vi "Data handler-Parameter Sweep.vi"(4 "Save image":bool, 5 "Save Ref image":bool, 6 "Single Frame Data":T2, 8 "error in (no error)":errorcluster, 9 "Live graph data queue in":T1, 10 "Logging queue element in":T5={"Imaging Protocol"=enum."Live Imaging", "Number of Trials"=0, "Frame Size"=512, "# Averaged frames"=0, "Dwell time (us)"=0.0, "Index of Z-plane"=0, "Timelapse?"=FALSE, "Logging process is active"=FALSE, "Speed logging enabled"=FALSE, "tdms file ref"=refnum, "path"=path "", "Trial Number"=0, "Expected # points acquired"=FALSE, "Manually stopped"=FALSE, "Last trial"=FALSE, "Ch0 data"=[], "Ch1 data"=[], "Ref Data"=[], "Ref Frame Time"=[], "Image Time"=[], "Continuous Time"=[], "Ref X Length"=0, "Ref Y Length"=0, "# Ref Averaged frames"=0, "Ref Dwell time (us)"=0.0, "Points acquired"={"Ch0 last trial"=0, "Ch1 last trial"=0, "All trials"=0}, "HW Timings File"=refnum} {"Ref Dwell time (us)" format="%#.6g"; "Frame Size" items=["100X100"=100, "128X128"=128, "200X200"=200, "256X256"=256, "512X512"=512, "1024x1024"=1024, "2048x2048"=2048]; "Dwell time (us)" format="%#.6g"}, 11 "Image array":T3) -> (0 "error out":errorcluster)   [LabVIEW 2017]
uses:
  Typedefs/Logging queue element.ctl
  Typedefs/Imaging Protocols enum.ctl
  Typedefs/Frame Size.ctl
  Typedefs/Acquired points count.ctl
  User Interface/Queue/Live graphs queue/Typedefs/Live imaging queue element.ctl
  <vilib>/vision/Image Controls.llb/IMAQ Image.ctl
  Typedefs/Frame data dual cluster.ctl
  User Interface/Typedefs/Live graph data queue ref.ctl
  Typedefs/fgv_actions.ctl
  Typedefs/Subpanel close request.ctl
  Typedefs/Top level VI states.ctl
  Typedefs/Channel Selector.ctl
  Global Variables/General Globals.vi
panel:
  out "Subpanel is closed / Proceed":bool
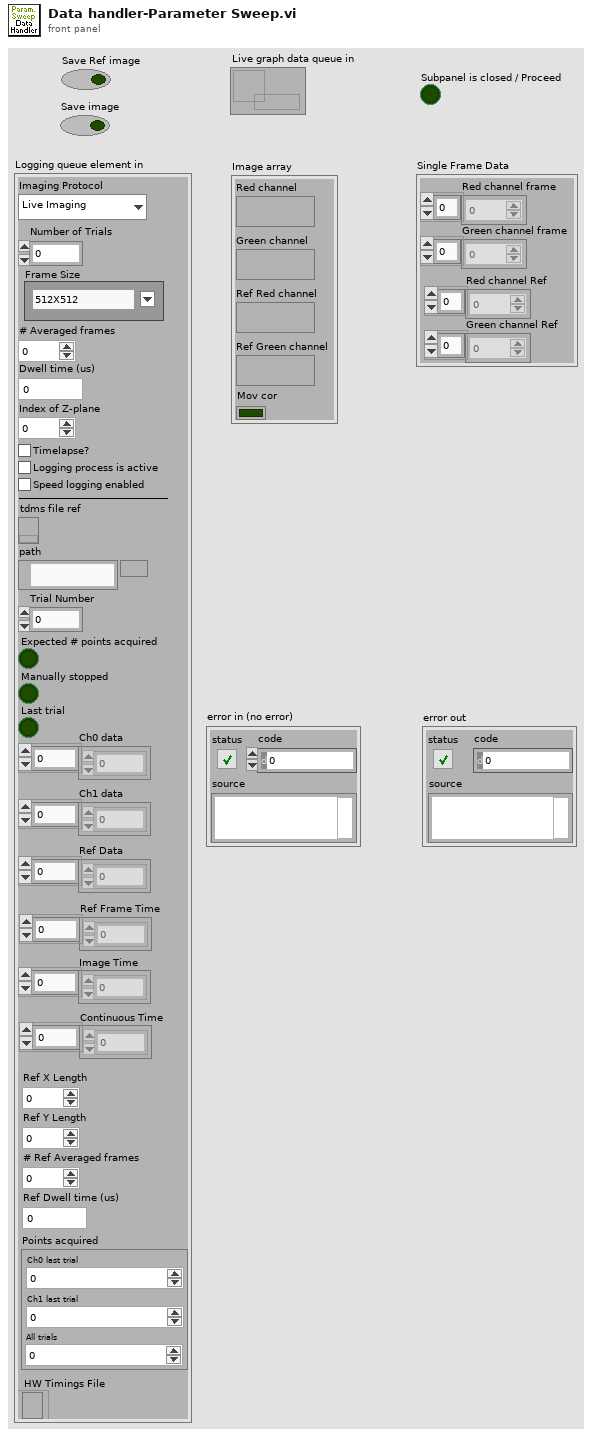
[diagram p1: front panel]
types:
  T1 = typedef "Live graph data queue ref.ctl" = refnum<queue>
  T2 = typedef "Frame data dual cluster.ctl" = cluster{"Red channel frame":dbl[], "Green channel frame":dbl[], "Red channel Ref":dbl[], "Green channel Ref":dbl[]}
  T3 = typedef "Live imaging queue element.ctl" = cluster{"Red channel":T4, "Green channel":T4, "Ref Red channel":T4, "Ref Green channel":T4, "Mov cor":bool}
  T4 = typedef "IMAQ Image.ctl" = refnum<image>
  T5 = typedef "Logging queue element.ctl" = cluster{"Imaging Protocol":T6, "Number of Trials":u16, "Frame Size":T7, "# Averaged frames":u16, "Dwell time (us)":dbl, "Index of Z-plane":i32, "Timelapse?":bool, "Logging process is active":bool, "Speed logging enabled":bool, "tdms file ref":refnum<k34>, "path":path, "Trial Number":i32, "Expected # points acquired":bool, "Manually stopped":bool, "Last trial":bool, "Ch0 data":u32[], "Ch1 data":u32[], "Ref Data":u32[], "Ref Frame Time":u64[], "Image Time":u64[], "Continuous Time":u64[], "Ref X Length":u16, "Ref Y Length":u16, "# Ref Averaged frames":u16, "Ref Dwell time (us)":dbl, "Points acquired":T8, "HW Timings File":refnum<file>}
  T6 = typedef "Imaging Protocols enum.ctl" = enum16{"AOL Z-Stack", "Motor Z Stack", "Parameter Sweep", "Functional Acquisition", "Single Plane Acquisition", "Volume Acquisition", "Live Imaging", "Live Plane Imaging", "Live Volume Imaging"}
  T7 = typedef "Frame Size.ctl" = u16
  T8 = typedef "Acquired points count.ctl" = cluster{"Ch0 last trial":u64, "Ch1 last trial":u64, "All trials":u64}
  T9 = typedef "fgv_actions.ctl" = enum16{"Get", "Set"}
  T10 = typedef "Subpanel close request.ctl" = enum16{"Request subpanel close", "Just check subpanel is closed"}
  T11 = typedef "Top level VI states.ctl" = enum16{"None", "Initialise UI", "<STACK PROTOCOL STATES>", "AOL Zstack-START", "AOL Zstack-STOP", "Motor Zstack-START", "Motor Zstack-STOP", "Parameter Sweep-START", "Parameter Sweep-STOP", "<ACQUISITION PROTOCOL STATES> ", "Functional Acquisition-START", "Functional Acquisition-STOP", "Single Plane Acquisition-START", "Single Plane Acquisition-STOP", "Volume Acquisition-START", "Volume Acquisition-STOP", "<LIVE IMAGING PROTOCOL STATES>", "Live Imaging-START", "Live Imaging-STOP", "Live Plane Imaging-START", "Live Plane Imaging-STOP", "Live Volume Imaging-START", "Live Volume Imaging-STOP", "<MOVEMENT CORRECTION PROTOCOL STATES>", "EXIT"}
  T12 = enum16{"open", "replace", "create", "open or create", "replace or create", "replace or create with confirmation"}
  T13 = typedef "Channel Selector.ctl" = enum16{"Red Channel", "Green Channel", "Blended"}
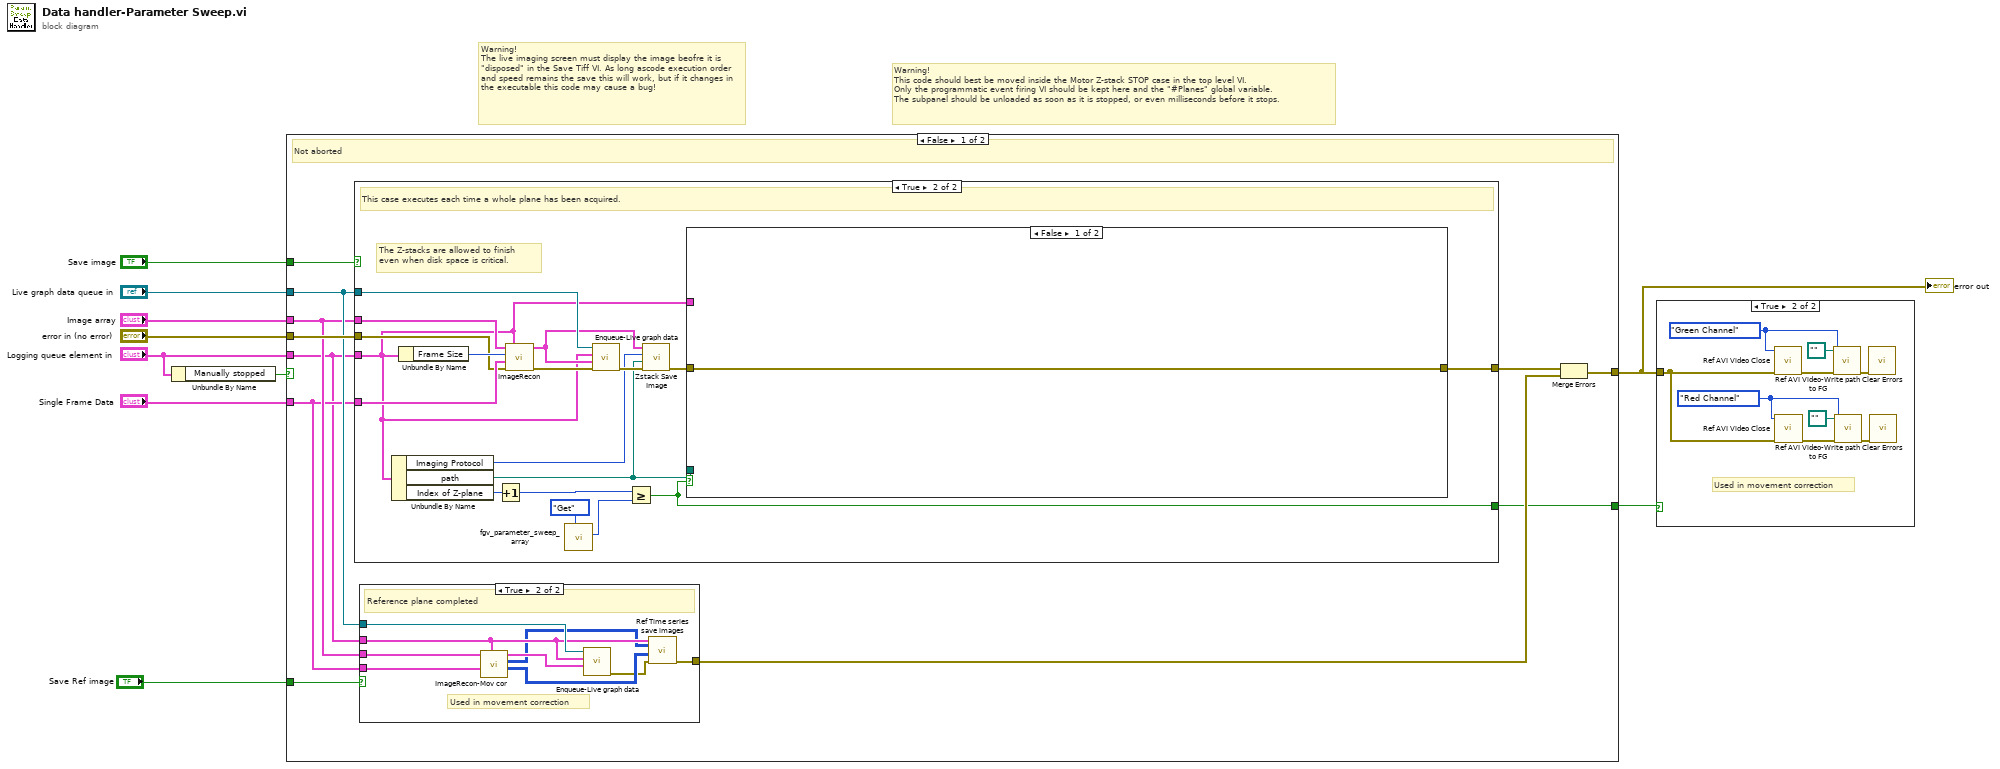
[diagram p0: block diagram]
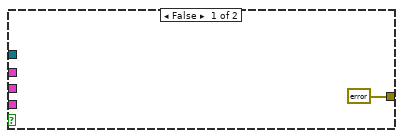
[diagram p2: hidden frame]
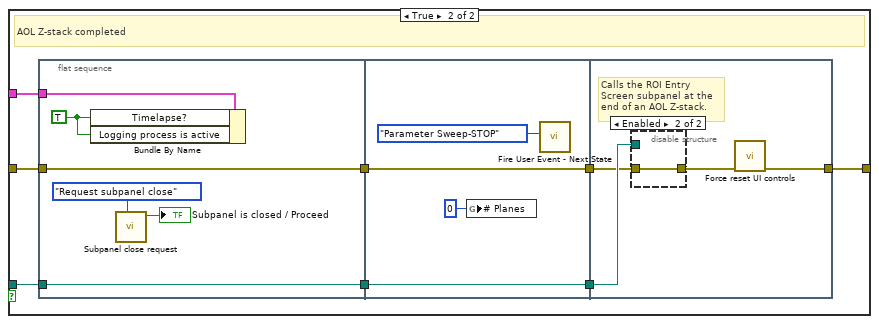
[diagram p4: hidden frame]
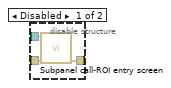
[diagram p5: hidden frame]
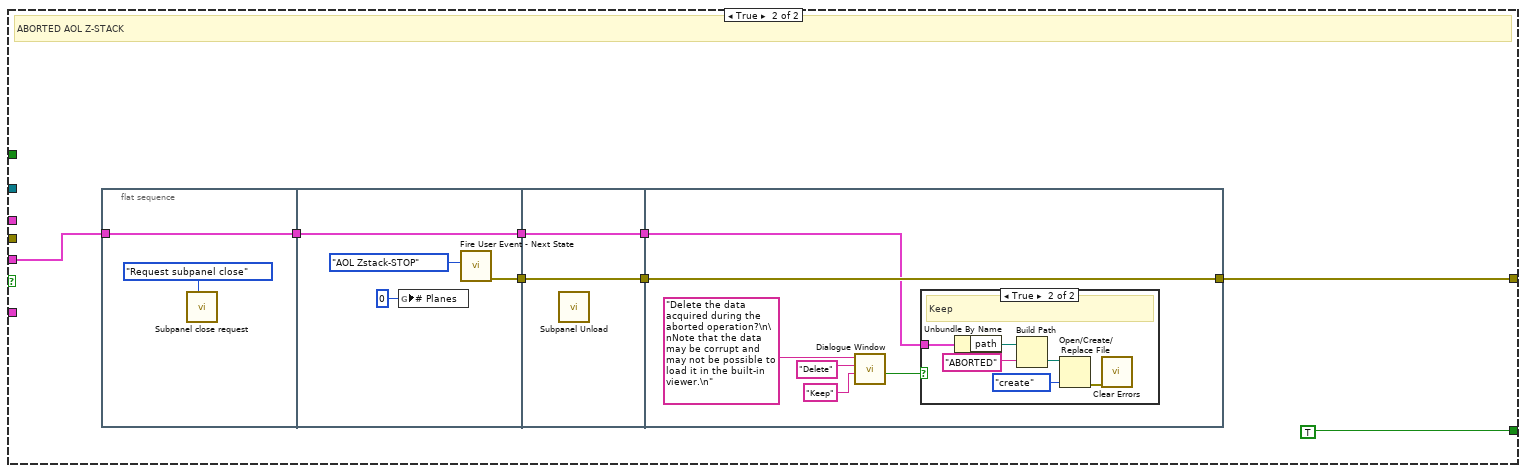
[diagram p6: hidden frame]
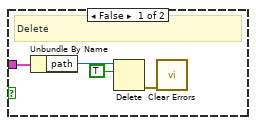
[diagram p7: hidden frame]
diagram:
  # "Warning!\nThe live imaging screen must display the image beofre it is \"disposed\" in the Save Tiff VI. As long ascode execution order and speed remains the save this will work, but if it changes in the executable this code may cause a bug!"
  # "Warning!\nThis code should best be moved inside the Motor Z-stack STOP case in the top level VI.\nOnly the programmatic event firing VI should be kept here and the \"#Planes\" global variable.\nThe subpanel should be unloaded as soon as it is stopped, or even milliseconds before it stops."
  n1 = Unbundle By Name("Logging queue element in") -> ("Manually stopped"=w1:bool)
  n2 = case shown="False" w1 {
    tunnel: "Save image" -> [w20 _]
    tunnel: "error in (no error)" -> [w19 _]
    tunnel: "Live graph data queue in" -> [w18 _]
    tunnel: "Image array" -> [w17 _]
    tunnel: "Single Frame Data" -> [w16 _]
    tunnel: [w14 w83] -> w5
    tunnel: "Save Ref image" -> [w13 _]
    tunnel: [w12 TRUE] -> w3
    tunnel: "Logging queue element in" -> [w11 w80]
    frame False {
      # "Not aborted"
      n3 = case shown="True" w20 {
        tunnel: [_ w49] -> w21
        tunnel: w17 -> [_ w47]
        tunnel: w11 -> [_ w36]
        tunnel: w16 -> [_ w44]
        tunnel: w19 -> [_ w43]
        tunnel: w18 -> [_ w42]
        tunnel: [_ w35] -> w12
        frame False {
          # "Acquisition of the current plane has not completed. Plane is incomplete."
        }
        frame True {
          # "The Z-stacks are allowed to finish even when disk space is critical."
          # "This case executes each time a whole plane has been acquired."
          n4 = Unbundle By Name(w36) -> ("Imaging Protocol"=w32:T6, "path"=w39:path, "Index of Z-plane"=w45:i32)
          n5 = Unbundle By Name(w36) -> ("Frame Size"=w46:T7)
          n6 = Increment(x=w45) -> (x+1=w48:i32)
          n7 = call "ImageRecon.vi"("Logging queue element in"=w36, "Error In"=w43, "Data"=w44, "Frame Size"=w46, "Image Array (in)"=w47) -> ("Error Out"=w38:errorcluster, "Image Array(out)"=w37:T3)  [unwired: 3 in, 2 out]
          n8 = call "fgv_parameter_sweep_array.vi"("FGV Actions"=fgv_actions."Get") -> ("Par. Sweep Array Size O/P"=w33:i32)  [unwired: 8 in, 2 out]
          n9 = call "Enqueue-Live graph data.vi"("error in (no error)"=w38, "Element to queue"=w37, "Logging queue element"=w36, "Live graph data queue in"=w42) -> ("error out"=w41:errorcluster)  [unwired: 6 in, 1 out]
          n10 = Greater Or Equal?(x=w48, y=w33) -> (x >= y?=w35:bool)
          n11 = call "Zstack Save Image.vi"("error in (no error)"=w41, "Dataset base-path"=w39, "Imaging Protocol"=w32, "Image Array"=w37) -> ("error out"=w40:errorcluster)  [unwired: 7 in]
          n12 = case shown="False" w35 {
            tunnel: w40 -> [w50 w56]
            tunnel: w39 -> [_ w58]
            tunnel: [w50 w57] -> w49
            tunnel: w36 -> [_ w51]
            frame False {
            }
            frame True {
              # "AOL Z-stack completed"
              n13 = flat-sequence {
                tunnel: w56 -> [w63]
                tunnel: w58 -> [w64]
                tunnel: [w64] -> w53
                tunnel: [w63] -> w52
                tunnel: w51 -> [w62]
                tunnel: [w68] -> w55
                tunnel: [w65] -> w54
                tunnel: w53 -> [w68]
                tunnel: w52 -> [w65]
                tunnel: [w69] -> w57
                tunnel: w55 -> [w72]
                tunnel: w54 -> [w71]
                frame #0 {
                  w61 = TRUE ("Timelapse?")
                  n14 = Bundle By Name(cluster=w62, "Timelapse?"=w61, "Logging process is active"=w61) -> ()  [unwired: 1 out]
                  n15 = call "Subpanel close request.vi"("Function"=Subpanel_close_request."Request subpanel close") -> ("Subpanel is closed / Proceed"=→"Subpanel is closed / Proceed":bool)  [unwired: 10 in]
                }
                frame #1 {
                  n16 = global write "General Globals.vi" "# Planes"(0 ("# Planes")) -> ()
                  n17 = call "Fire User Event - Next State.vi"("\"UI Handler loop\" case to execute"=Top_level_VI_states."Parameter Sweep-STOP" ("event data / imaging mode")) -> ()  [unwired: 10 in, 1 out]
                }
                frame #2 {
                  # "Calls the ROI Entry Screen subpanel at the end of an AOL Z-stack."
                  n18 = disable-structure shown="Enabled" {
                    disable-tunnel: w72 -> [w75 _]
                    disable-tunnel: [w74 w76] -> w70
                    disable-tunnel: w71 -> [w73 w76]
                    frame Disabled {
                      n19 = call "Subpanel call-ROI entry screen.vi"("error in"=w73, "Experiment folder path"=w75) -> ("error out"=w74:errorcluster)  [unwired: 9 in]
                    }
                    frame Enabled {
                    }
                  }
                  n20 = call "Force reset UI controls.vi"("error in (no error)"=w70) -> ("error out"=w69:errorcluster)  [unwired: 10 in]
                }
              }
            }
          }
        }
      }
      n21 = case shown="True" w13 {
        tunnel: w11 -> [_ w28]
        tunnel: [errorcluster {"status"=FALSE, "code"=0, "source"=""} ("error out") w31] -> w15
        tunnel: w18 -> [_ w30]
        tunnel: w17 -> [_ w29]
        tunnel: w16 -> [_ w26]
        frame False {
        }
        frame True {
          # "Used in movement correction"
          # "Reference plane completed"
          n22 = call "ImageRecon-Mov cor.vi"("Logging queue element in"=w28, "Data"=w26, "Image Array (in)"=w29) -> ("Ch1-Green-REF"=w24:i16[][], "Ch0-Red-REF"=w25:i16[][], "Image Array(out)"=w27:T3)  [unwired: 5 in, 1 out]
          n23 = call "Enqueue-Live graph data.vi"("Element to queue"=w27, "Logging queue element"=w28, "Live graph data queue in"=w30) -> ("error out"=w23:errorcluster)  [unwired: 7 in, 1 out]
          n24 = call "Ref Time series save images.vi"("error in (no error)"=w23, "Ch1-Green-REF"=w24, "Ch0-Red-REF"=w25, "Logging queue element"=w28) -> ("error"=w31:errorcluster)  [unwired: 7 in]
        }
      }
      n25 = Merge Errors(w21, w15) -> (w14:errorcluster)
    }
    frame True {
      # "ABORTED AOL Z-STACK"
      n26 = flat-sequence {
        tunnel: w80 -> [w85]
        tunnel: [w85] -> w79
        tunnel: [w88] -> w82
        tunnel: w79 -> [w87]
        tunnel: [w87] -> w78
        tunnel: w82 -> [w92]
        tunnel: [w92] -> w81
        tunnel: w78 -> [w91]
        tunnel: [w91] -> w77
        tunnel: [w98] -> w83
        tunnel: w81 -> [w98]
        tunnel: w77 -> [w94]
        frame #0 {
          n27 = call "Subpanel close request.vi"("Function"=Subpanel_close_request."Request subpanel close") -> ()  [unwired: 10 in, 1 out]
        }
        frame #1 {
          n28 = global write "General Globals.vi" "# Planes"(0 ("# Planes")) -> ()
          n29 = call "Fire User Event - Next State.vi"("\"UI Handler loop\" case to execute"=Top_level_VI_states."AOL Zstack-STOP" ("event data / imaging mode")) -> ("Error Out"=w88:errorcluster)  [unwired: 10 in]
        }
        frame #2 {
          n30 = call "Subpanel Unload.vi"() -> ()  [unwired: 11 in, 1 out]
        }
        frame #3 {
          n31 = call "Dialogue Window.vi"("Caption-Left button (Cancel)"="Keep", "Caption-Right button (OK)"="Delete", "Message string"="Delete the data acquired during the aborted operation?\n\nNote that the data may be corrupt and may not be possible to load it in the built-in viewer.\n") -> ("Cancelled (Left button pressed)"=w95:bool)  [unwired: 6 in, 2 out]
          n32 = case shown="True" w95 {
            tunnel: w94 -> [w102 w103]
            frame False {
              # "Delete"
              n33 = Unbundle By Name(w102) -> ("path"=w101:path)
              n34 = Delete(path (use dialog)=w101, entire hierarchy (F)=TRUE) -> (error out=w99:errorcluster)  [unwired: 3 in, 2 out]
              n35 = call <vilib>:"Clear Errors.vi"("error in (no error)"=w99) -> ()  [unwired: 5 in, 2 out]
            }
            frame True {
              # "Keep"
              n36 = Unbundle By Name(w103) -> ("path"=w108:path)
              n37 = Build Path(base path=w108, name or relative path="ABORTED") -> (appended path=w105:path)
              n38 = Open/Create/Replace File(file path (use dialog)=w105, operation (0:open)=T12."create") -> (error out=w107:errorcluster)  [unwired: 4 in, 2 out]
              n39 = call <vilib>:"Clear Errors.vi"("error in (no error)"=w107) -> ()  [unwired: 5 in, 2 out]
            }
          }
        }
      }
    }
  }
  "error out" <- w5
  n40 = case shown="True" w3 {
    tunnel: w5 -> [_ w111]
    frame False {
    }
    frame True {
      w109 = Channel_Selector."Red Channel" ("Channel")
      w110 = Channel_Selector."Green Channel" ("Channel")
      # "Used in movement correction"
      n41 = call "Ref AVI Video Close.vi"("error in (no error)"=w111, "Channel"=w110) -> ("error out"=w117:errorcluster)  [unwired: 9 in]
      n42 = call "Ref AVI Video Close.vi"("error in (no error)"=w111, "Channel"=w109) -> ("error out"=w112:errorcluster)  [unwired: 9 in]
      n43 = call "Ref AVI Video-Write path to FG.vi"("error in (no error)"=w117, "Channel"=w110, "AVI2 path"=path "") -> ("error out"=w115:errorcluster)  [unwired: 8 in]
      n44 = call "Ref AVI Video-Write path to FG.vi"("error in (no error)"=w112, "Channel"=w109, "AVI2 path"=path "") -> ("error out"=w114:errorcluster)  [unwired: 8 in]
      n45 = call <vilib>:"Clear Errors.vi"("error in (no error)"=w115) -> ()  [unwired: 5 in, 2 out]
      n46 = call <vilib>:"Clear Errors.vi"("error in (no error)"=w114) -> ()  [unwired: 5 in, 2 out]
    }
  }
